vi "Intaris_USB_Build bmRequestType.vi"(4 "bmRequest Parameters":T1) -> (1 "bmRequest":i16 format="Dec : %.0f\nHex : %x\nBin : %08b")   [LabVIEW 2014]
uses:
  bmRequestType_direction.ctl
  bmRequestType_type.ctl
  bmRequestType_recipient.ctl
  bmRequestType Parameters.ctl
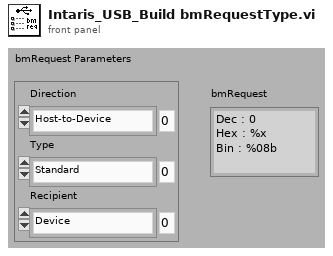
[diagram p1: front panel]
types:
  T1 = typedef "bmRequestType Parameters.ctl" = cluster{"Direction":T2, "Type":T3, "Recipient":T4}
  T2 = typedef "bmRequestType_direction.ctl" = enum16{"Host-to-Device", "Device-to-Host"}
  T3 = typedef "bmRequestType_type.ctl" = enum16{"Standard", "Class", "Vendor"}
  T4 = typedef "bmRequestType_recipient.ctl" = enum16{"Device", "Interface", "Endpoint", "Other"}
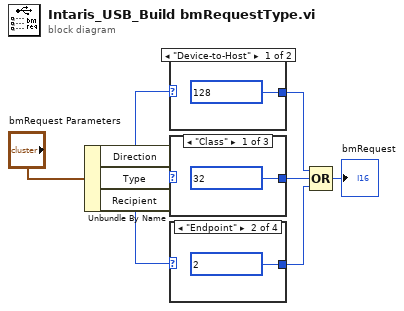
[diagram p0: block diagram]
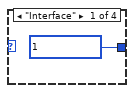
[diagram p2: hidden frame]
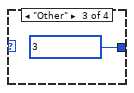
[diagram p3: hidden frame]
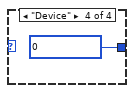
[diagram p4: hidden frame]
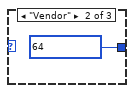
[diagram p5: hidden frame]
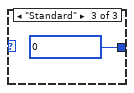
[diagram p6: hidden frame]
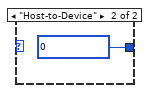
[diagram p7: hidden frame]
diagram:
  n1 = Unbundle By Name("bmRequest Parameters") -> ("Direction"=w3:T2, "Type"=w2:T3, "Recipient"=w1:T4)
  n2 = case shown="\"Device-to-Host\"" w3 {
    tunnel: [i16 128 i16 0] -> w8
    frame "Device-to-Host" {
    }
    frame "Host-to-Device" {
    }
  }
  n3 = case shown="\"Class\"" w2 {
    tunnel: [i16 32 i16 64 i16 0] -> w6
    frame "Class" {
    }
    frame "Vendor" {
    }
    frame "Standard" {
    }
  }
  n4 = case shown="\"Endpoint\"" w1 {
    tunnel: [i16 1 i16 2 i16 3 i16 0] -> w7
    frame "Interface" {
    }
    frame "Endpoint" {
    }
    frame "Other" {
    }
    frame "Device" {
    }
  }
  n5 = Compound Arithmetic op=OR(w8, w6, w7) -> (→"bmRequest":i16)
